vi "Control Operations.vi"(8 "error in (no error)":errorcluster, 9 "Value":i32, 10 "Command":T1, 11 "VISA resource name":refnum<visa-resource-name>) -> (0 "error out":errorcluster, 3 "VISA resource name out":refnum<visa-resource-name>)   [LabVIEW 2020, in "Jasco UV.lvlib"]
uses:
  Jasco UV.lvlib
  Operations.ctl
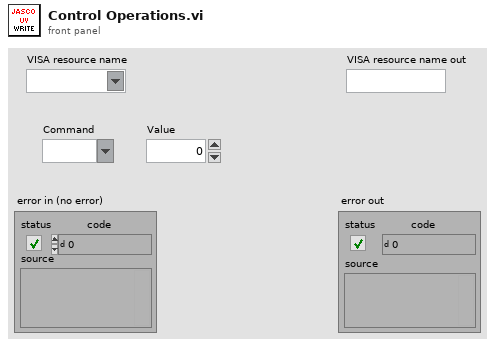
[diagram p1: front panel]
types:
  T1 = typedef "Jasco UV.lvlib/Operations.ctl" = string
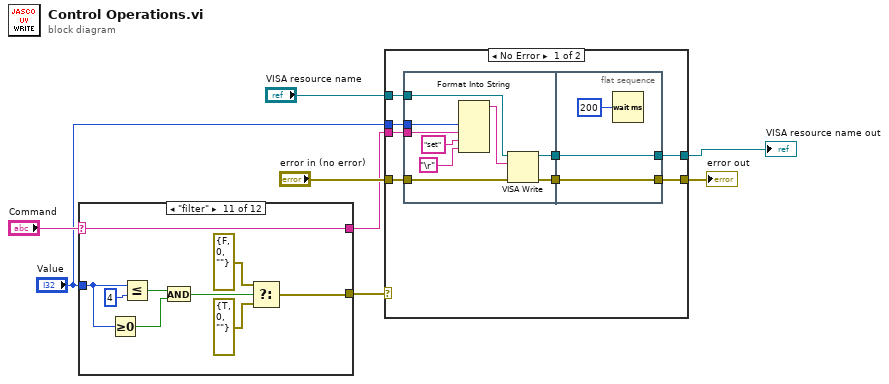
[diagram p0: block diagram]
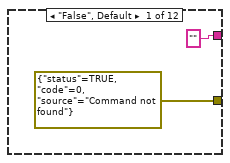
[diagram p3: hidden frame]
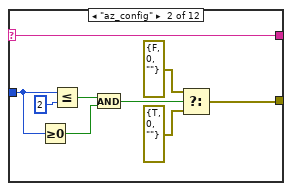
[diagram p4: hidden frame]
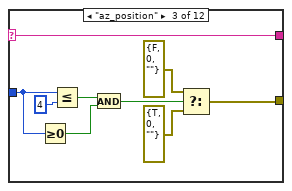
[diagram p5: hidden frame]
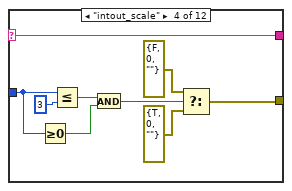
[diagram p6: hidden frame]
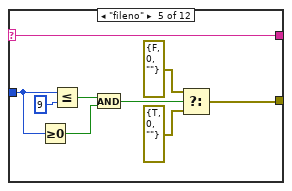
[diagram p7: hidden frame]
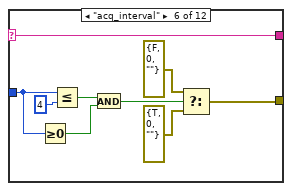
[diagram p8: hidden frame]
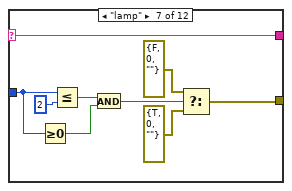
[diagram p9: hidden frame]
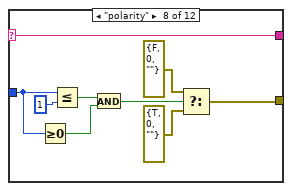
[diagram p10: hidden frame]
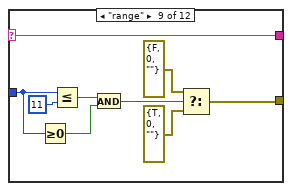
[diagram p11: hidden frame]
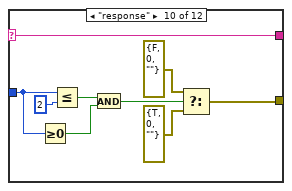
[diagram p12: hidden frame]
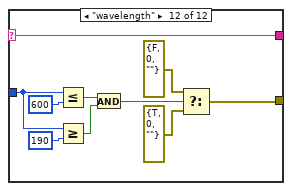
[diagram p13: hidden frame]
diagram:
  n1 = case shown="\"filter\"" "Command" {
    selector: "Command" -> [_ w19 w28 w37 w46 w55 w64 w73 w82 w91 w100 w110]
    tunnel: ["" w19 w28 w37 w46 w55 w64 w73 w82 w91 w100 w110] -> w3
    tunnel: "Value" -> [_ w18 w27 w36 w45 w54 w63 w72 w81 w90 w99 w102]
    tunnel: [errorcluster {"status"=TRUE, "code"=0, "source"="Command not found"} ("error in (no error)") w11 w20 w29 w38 w47 w56 w65 w74 w83 w92 w103] -> w2
    frame "False", Default {
    }
    frame "az_config" {
      n2 = Greater Or Equal To 0?(x=w18) -> (x >= 0?=w15:bool)
      n3 = Less Or Equal?(x=w18, y=2) -> (x <= y?=w16:bool)
      n4 = And(x=w16, y=w15) -> (x .and. y?=w14:bool)
      n5 = Select(t=errorcluster {"status"=FALSE, "code"=0, "source"=""} ("error in (no error)"), s=w14, f=errorcluster {"status"=TRUE, "code"=0, "source"=""} ("error in (no error)")) -> (s? t:f=w11:errorcluster)
    }
    frame "az_position" {
      n6 = Greater Or Equal To 0?(x=w27) -> (x >= 0?=w24:bool)
      n7 = Less Or Equal?(x=w27, y=4) -> (x <= y?=w25:bool)
      n8 = And(x=w25, y=w24) -> (x .and. y?=w23:bool)
      n9 = Select(t=errorcluster {"status"=FALSE, "code"=0, "source"=""} ("error in (no error)"), s=w23, f=errorcluster {"status"=TRUE, "code"=0, "source"=""} ("error in (no error)")) -> (s? t:f=w20:errorcluster)
    }
    frame "intout_scale" {
      n10 = Greater Or Equal To 0?(x=w36) -> (x >= 0?=w33:bool)
      n11 = Less Or Equal?(x=w36, y=3) -> (x <= y?=w34:bool)
      n12 = And(x=w34, y=w33) -> (x .and. y?=w32:bool)
      n13 = Select(t=errorcluster {"status"=FALSE, "code"=0, "source"=""} ("error in (no error)"), s=w32, f=errorcluster {"status"=TRUE, "code"=0, "source"=""} ("error in (no error)")) -> (s? t:f=w29:errorcluster)
    }
    frame "fileno" {
      n14 = Greater Or Equal To 0?(x=w45) -> (x >= 0?=w42:bool)
      n15 = Less Or Equal?(x=w45, y=9) -> (x <= y?=w43:bool)
      n16 = And(x=w43, y=w42) -> (x .and. y?=w41:bool)
      n17 = Select(t=errorcluster {"status"=FALSE, "code"=0, "source"=""} ("error in (no error)"), s=w41, f=errorcluster {"status"=TRUE, "code"=0, "source"=""} ("error in (no error)")) -> (s? t:f=w38:errorcluster)
    }
    frame "acq_interval" {
      n18 = Greater Or Equal To 0?(x=w54) -> (x >= 0?=w51:bool)
      n19 = Less Or Equal?(x=w54, y=4) -> (x <= y?=w52:bool)
      n20 = And(x=w52, y=w51) -> (x .and. y?=w50:bool)
      n21 = Select(t=errorcluster {"status"=FALSE, "code"=0, "source"=""} ("error in (no error)"), s=w50, f=errorcluster {"status"=TRUE, "code"=0, "source"=""} ("error in (no error)")) -> (s? t:f=w47:errorcluster)
    }
    frame "lamp" {
      n22 = Greater Or Equal To 0?(x=w63) -> (x >= 0?=w60:bool)
      n23 = Less Or Equal?(x=w63, y=2) -> (x <= y?=w61:bool)
      n24 = And(x=w61, y=w60) -> (x .and. y?=w59:bool)
      n25 = Select(t=errorcluster {"status"=FALSE, "code"=0, "source"=""} ("error in (no error)"), s=w59, f=errorcluster {"status"=TRUE, "code"=0, "source"=""} ("error in (no error)")) -> (s? t:f=w56:errorcluster)
    }
    frame "polarity" {
      n26 = Greater Or Equal To 0?(x=w72) -> (x >= 0?=w69:bool)
      n27 = Less Or Equal?(x=w72, y=1) -> (x <= y?=w70:bool)
      n28 = And(x=w70, y=w69) -> (x .and. y?=w68:bool)
      n29 = Select(t=errorcluster {"status"=FALSE, "code"=0, "source"=""} ("error in (no error)"), s=w68, f=errorcluster {"status"=TRUE, "code"=0, "source"=""} ("error in (no error)")) -> (s? t:f=w65:errorcluster)
    }
    frame "range" {
      n30 = Greater Or Equal To 0?(x=w81) -> (x >= 0?=w78:bool)
      n31 = Less Or Equal?(x=w81, y=11) -> (x <= y?=w79:bool)
      n32 = And(x=w79, y=w78) -> (x .and. y?=w77:bool)
      n33 = Select(t=errorcluster {"status"=FALSE, "code"=0, "source"=""} ("error in (no error)"), s=w77, f=errorcluster {"status"=TRUE, "code"=0, "source"=""} ("error in (no error)")) -> (s? t:f=w74:errorcluster)
    }
    frame "response" {
      n34 = Greater Or Equal To 0?(x=w90) -> (x >= 0?=w87:bool)
      n35 = Less Or Equal?(x=w90, y=2) -> (x <= y?=w88:bool)
      n36 = And(x=w88, y=w87) -> (x .and. y?=w86:bool)
      n37 = Select(t=errorcluster {"status"=FALSE, "code"=0, "source"=""} ("error in (no error)"), s=w86, f=errorcluster {"status"=TRUE, "code"=0, "source"=""} ("error in (no error)")) -> (s? t:f=w83:errorcluster)
    }
    frame "filter" {
      n38 = Greater Or Equal To 0?(x=w99) -> (x >= 0?=w96:bool)
      n39 = Less Or Equal?(x=w99, y=4) -> (x <= y?=w97:bool)
      n40 = And(x=w97, y=w96) -> (x .and. y?=w95:bool)
      n41 = Select(t=errorcluster {"status"=FALSE, "code"=0, "source"=""} ("error in (no error)"), s=w95, f=errorcluster {"status"=TRUE, "code"=0, "source"=""} ("error in (no error)")) -> (s? t:f=w92:errorcluster)
    }
    frame "wavelength" {
      n42 = Less Or Equal?(x=w102, y=600) -> (x <= y?=w108:bool)
      n43 = Greater Or Equal?(x=w102, y=190) -> (x >= y?=w107:bool)
      n44 = And(x=w108, y=w107) -> (x .and. y?=w106:bool)
      n45 = Select(t=errorcluster {"status"=FALSE, "code"=0, "source"=""} ("error in (no error)"), s=w106, f=errorcluster {"status"=TRUE, "code"=0, "source"=""} ("error in (no error)")) -> (s? t:f=w103:errorcluster)
    }
  }
  n46 = case shown="No Error" w2 {
    tunnel: "VISA resource name" -> [w116 w131]
    tunnel: [w115 w131] -> w7
    tunnel: [w114 w132] -> w6
    tunnel: "error in (no error)" -> [w113 w132]
    tunnel: w3 -> [w112 _]
    tunnel: "Value" -> [w111 _]
    frame No Error {
      n47 = flat-sequence {
        tunnel: w112 -> [w120]
        tunnel: w113 -> [w127]
        tunnel: w116 -> [w126]
        tunnel: [w125] -> w118
        tunnel: [w124] -> w117
        tunnel: w111 -> [w119]
        tunnel: [w129] -> w114
        tunnel: w118 -> [w129]
        tunnel: [w128] -> w115
        tunnel: w117 -> [w128]
        frame #0 {
          n48 = Format Into String(w119, w120, "set" ("string"), "\r") -> (resulting string=w121:string)  [unwired: 3 in, 1 out]
          n49 = VISA Write(VISA resource name=w126, write buffer=w121, error in (no error)=w127) -> (VISA resource name out=w124:refnum<visa-resource-name>, error out=w125:errorcluster)  [unwired: 1 out]
        }
        frame #1 {
          n50 = Wait (ms)(milliseconds to wait=u32 200) -> ()  [unwired: 1 out]
        }
      }
    }
    frame Error {
    }
  }
  "VISA resource name out" <- w7
  "error out" <- w6
